vi "MotorCommand.vi"() -> ()   [LabVIEW 2010]
panel:
  out "Value 8":u16=1000
  in  "Enable 8":bool
  in  "Motor 8":u16(slide)=1000 min=1000 max=2000 scale=1000.0..2000.0
  out "Value 7":u16=1000
  in  "Enable 7":bool
  in  "Motor 7":u16(slide)=1000 min=1000 max=2000 scale=1000.0..2000.0
  out "Value 6":u16=1000
  in  "Enable 6":bool
  in  "Motor 6":u16(slide)=1000 min=1000 max=2000 scale=1000.0..2000.0
  out "Value 5":u16=1000
  in  "Enable 5":bool
  in  "Motor 5":u16(slide)=1000 min=1000 max=2000 scale=1000.0..2000.0
  out "Value 4":u16=1000
  in  "Enable 4":bool
  in  "Motor 4":u16(slide)=1000 min=1000 max=2000 scale=1000.0..2000.0
  out "Value 3":u16=1000
  in  "Enable 3":bool
  in  "Motor 3":u16(slide)=1000 min=1000 max=2000 scale=1000.0..2000.0
  out "Value 2":u16=1000
  in  "Enable 2":bool
  in  "Motor 2":u16(slide)=1000 min=1000 max=2000 scale=1000.0..2000.0
  out "Value 1":u16=1000
  in  "Enable 1":bool
  in  "Motor 1":u16(slide)=1000 min=1000 max=2000 scale=1000.0..2000.0
  in  "SendCommand":bool
  in  "StopCommand":bool
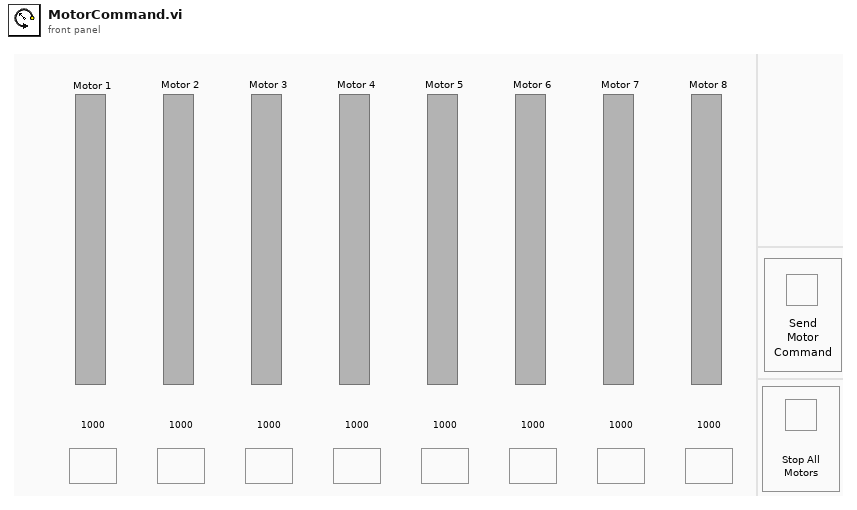
[diagram p1: front panel]
types:
  T1 = cluster{"Error":errorcluster, "GUIQueue":refnum<queue>, "TlmType":string, "NextState":string, "MotorCount":i32, "IniData":string[][]}
  T2 = enum8{"Enabled", "Disabled", "Disabled and Grayed Out"}
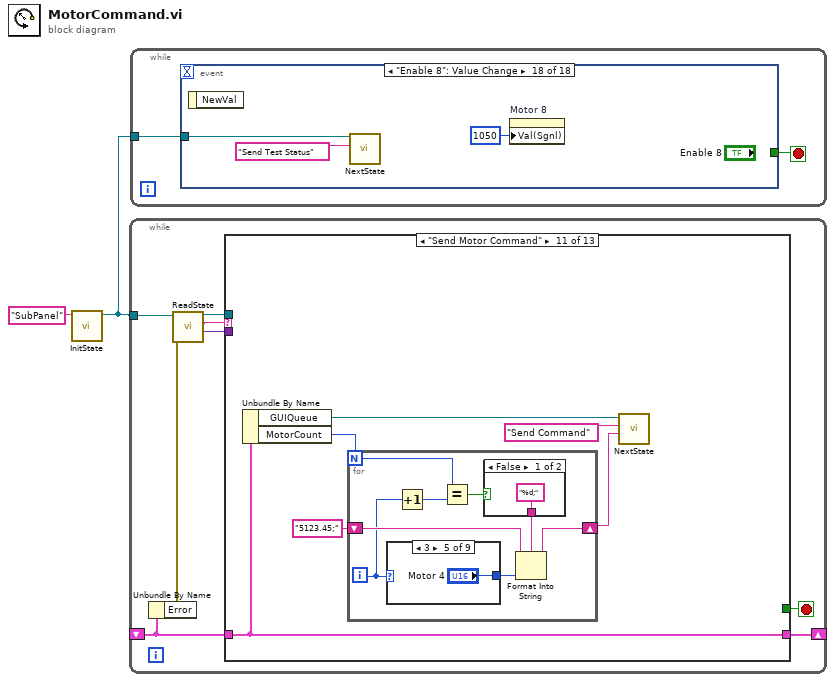
[diagram p0: block diagram]
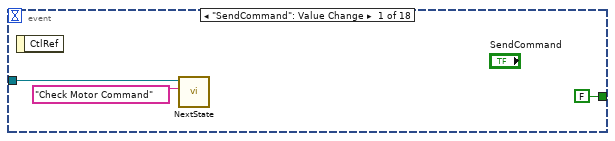
[diagram p2: hidden frame]
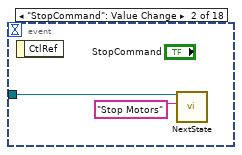
[diagram p3: hidden frame]
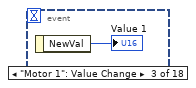
[diagram p4: hidden frame]
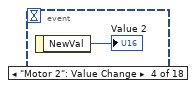
[diagram p5: hidden frame]
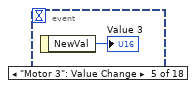
[diagram p6: hidden frame]
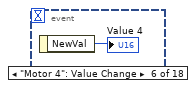
[diagram p7: hidden frame]
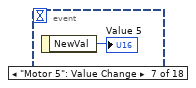
[diagram p8: hidden frame]
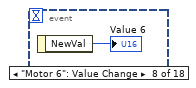
[diagram p9: hidden frame]
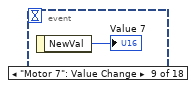
[diagram p10: hidden frame]
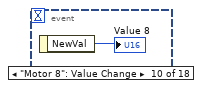
[diagram p11: hidden frame]
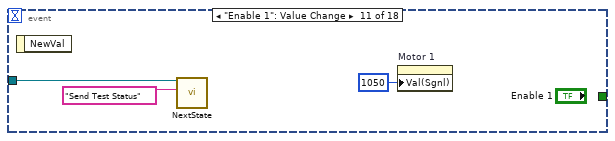
[diagram p12: hidden frame]
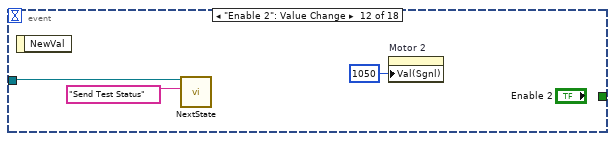
[diagram p13: hidden frame]
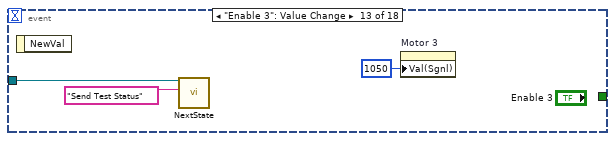
[diagram p14: hidden frame]
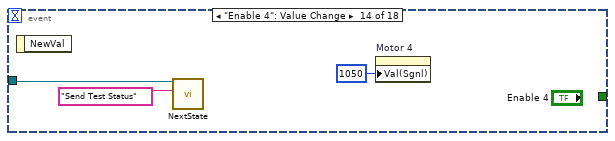
[diagram p15: hidden frame]
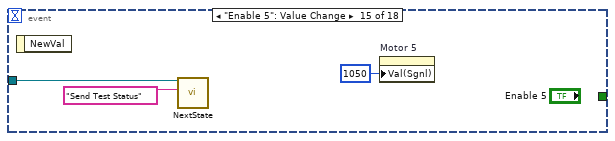
[diagram p16: hidden frame]
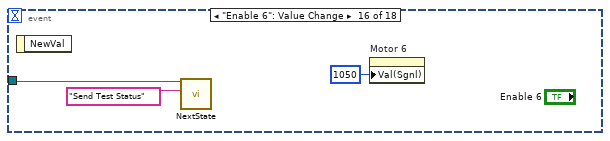
[diagram p17: hidden frame]
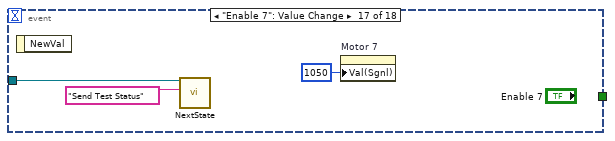
[diagram p18: hidden frame]
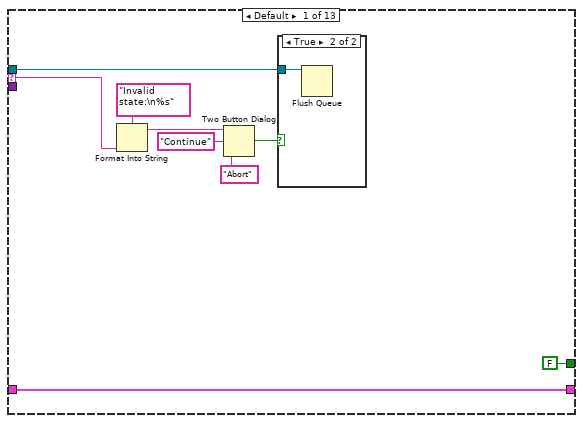
[diagram p19: hidden frame]
diagram:
  n1 = call "InitState.vi"("Name"="SubPanel" ("name (unnamed)")) -> ("Queue Out"=w1:refnum<queue>)  [unwired: 8 in, 1 out]
  n2 = while {
    tunnel: w1 -> [w7]
    shift-right: [w10] -> _
    shift-left: _ -> [w9]
    stop <- w8 stop-if-true
    n3 = Unbundle By Name(w9) -> ("Error"=w6:errorcluster)
    n4 = call "ReadState.vi"("Error In"=w6, "Queue In"=w7) -> ("Data"=w5:variant, "State"=w4:string, "Queue Out"=w3:refnum<queue>)  [unwired: 6 in, 1 out]
    n5 = case shown="\"Send Motor Command\"" w4 {
      tunnel: w3 -> [w11 _ w26 w35 _ _ _ _ _ w78 _ _ w135]
      selector: w4 -> [w17 _ _ _ _ _ _ _ _ _ _ _ _]
      tunnel: w5 -> [_ _ w27 _ _ w70 _ _ _ _ _ _ _]
      tunnel: [w16 w23 w32 w38 w52 w69 w72 w74 w75 w91 w108 w127 w132] -> w10
      tunnel: w9 -> [w16 w23 _ w39 w52 w69 w72 w74 w75 w91 w108 w127 w132]
      tunnel: [FALSE TRUE _ _ _ _ _ TRUE _ _ _ _ _] -> w8
      frame Default {
        n6 = Format Into String(format string="Invalid state:\n%s", w17) -> (resulting string=w18:string)  [unwired: 2 in, 1 out]
        n7 = Two Button Dialog(message=w18, 1:"Abort" ("F button name (\"Cancel\")"), 2:"Continue" ("T button name (\"OK\")")) -> (T button?=w12:bool)
        n8 = case shown="True" w12 {
          tunnel: w11 -> [_ w20]
          frame False {
          }
          frame True {
            n9 = Flush Queue(queue=w20) -> ()  [unwired: 1 in, 3 out]
          }
        }
      }
      frame "Error" {
        n10 = Unbundle By Name(w23) -> ("Error"=w22:errorcluster)
        n11 = call "ErrorDialog.vi"("error in"=w22) -> ("error out"=w21:errorcluster)  [unwired: 10 in]
        n12 = call <vilib>:"Clear Errors.vi"("error in (no error)"=w21) -> ()  [unwired: 6 in, 1 out]
      }
      frame "Initialize" {
        n13 = call "NextState.vi"("State"="Read Initialization", "Queue In"=w26) -> ()  [unwired: 8 in, 2 out]
        n14 = Variant To Data(Variant=w27, type=string[][] [] ("subarray")) -> (data=w29:string[][])  [unwired: 1 in, 1 out]
        n15 = call "InitState.vi"("Name"="GUI") -> ("Queue Out"=w28:refnum<queue>)  [unwired: 8 in, 1 out]
        n16 = Bundle By Name(cluster=T1 {"Error"={"status"=FALSE, "code"=0, "source"=""}, "GUIQueue"=refnum, "TlmType"="", "NextState"="", "MotorCount"=0, "IniData"=[]}, "IniData"=w29, "GUIQueue"=w28) -> (w32:T1)
      }
      frame "Read Initialization" {
        n17 = Unbundle By Name(w39) -> ("IniData"=w41:string[][])
        n18 = call "NextState.vi"("State"="Update Motor Count", "Queue In"=w35) -> ()  [unwired: 8 in, 2 out]
        n19 = Index Array(array=w41, index (col)=0 ("index (row)")) -> (element=w43:string[])  [unwired: 1 in]
        n20 = for {
          tunnel: w43 -> [w50]
          tunnel: string[] ["Motors"] -> [w46] mode=indexing
          tunnel: w41 -> [w49]
          tunnel: [w45] -> w40 mode=indexing
          n21 = Search 1D Array(1D array=w50, element=w46) -> (index of element=w47:i32)  [unwired: 1 in]
          n22 = Index Array(array=w49, index (row)=w47, index (col)=1 ("disabled index (col)")) -> (element=w45:string)
        }
        n23 = Index Array(array=w40) -> (element=w37:string)  [unwired: 1 in]
        n24 = Decimal String To Number(string=w37) -> (number=w36:i32)  [unwired: 2 in, 1 out]
        n25 = Bundle By Name(cluster=w39, "MotorCount"=w36) -> (w38:T1)
      }
      frame "Update Motor Count" {
        n26 = Unbundle By Name(w52) -> ("MotorCount"=w51:i32)
        n27 = for {
          N: 8 -> [_]
          tunnel: w51 -> [w55]
          i -> [w54]
          n28 = Less?(x=w54, y=w55) -> (x < y?=w59:bool)
          n29 = Select(t=T2."Enabled" ("Disabled"), s=w59, f=T2."Disabled and Grayed Out" ("Disabled")) -> (s? t:f=w58:T2)
          n30 = case shown="0" w54 {
            tunnel: w58 -> [_ w60 w61 w62 w63 w64 w65 w66 w67]
            frame Default {
            }
            frame 0 {
              n31 = property on="Motor 1" class="Slide (strict)"("DisabledEnum"=w60) -> ()  [unwired: 2 in, 2 out]
              n32 = property on="Enable 1" class="Bool"("DisabledEnum"=w60) -> ()  [unwired: 2 in, 2 out]
            }
            frame 1 {
              n33 = property on="Motor 2" class="Slide (strict)"("DisabledEnum"=w61) -> ()  [unwired: 2 in, 2 out]
              n34 = property on="Enable 2" class="Bool"("DisabledEnum"=w61) -> ()  [unwired: 2 in, 2 out]
            }
            frame 2 {
              n35 = property on="Motor 3" class="Slide (strict)"("DisabledEnum"=w62) -> ()  [unwired: 2 in, 2 out]
              n36 = property on="Enable 3" class="Bool"("DisabledEnum"=w62) -> ()  [unwired: 2 in, 2 out]
            }
            frame 3 {
              n37 = property on="Motor 4" class="Slide (strict)"("DisabledEnum"=w63) -> ()  [unwired: 2 in, 2 out]
              n38 = property on="Enable 4" class="Bool"("DisabledEnum"=w63) -> ()  [unwired: 2 in, 2 out]
            }
            frame 4 {
              n39 = property on="Motor 5" class="Slide (strict)"("DisabledEnum"=w64) -> ()  [unwired: 2 in, 2 out]
              n40 = property on="Enable 5" class="Bool"("DisabledEnum"=w64) -> ()  [unwired: 2 in, 2 out]
            }
            frame 5 {
              n41 = property on="Motor 6" class="Slide (strict)"("DisabledEnum"=w65) -> ()  [unwired: 2 in, 2 out]
              n42 = property on="Enable 6" class="Bool"("DisabledEnum"=w65) -> ()  [unwired: 2 in, 2 out]
            }
            frame 6 {
              n43 = property on="Motor 7" class="Slide (strict)"("DisabledEnum"=w66) -> ()  [unwired: 2 in, 2 out]
              n44 = property on="Enable 7" class="Bool"("DisabledEnum"=w66) -> ()  [unwired: 2 in, 2 out]
            }
            frame 7 {
              n45 = property on="Motor 8" class="Slide (strict)"("DisabledEnum"=w67) -> ()  [unwired: 2 in, 2 out]
              n46 = property on="Enable 8" class="Bool"("DisabledEnum"=w67) -> ()  [unwired: 2 in, 2 out]
            }
          }
        }
      }
      frame "Update" {
        n47 = Variant To Data(Variant=w70, type=dbl[][] []) -> ()  [unwired: 1 in, 2 out]
      }
      frame "Temporary" {
        n48 = One Button Dialog(message="This feature under contruction.") -> ()  [unwired: 1 in, 1 out]
      }
      frame "Shutdown" {
      }
      frame "----------" {
      }
      frame "Check Motor Command" {
        n49 = local read "Motor 1"() -> (w90:u16)
        n50 = local read "Motor 2"() -> (w89:u16)
        n51 = local read "Motor 3"() -> (w88:u16)
        n52 = local read "Motor 4"() -> (w87:u16)
        n53 = local read "Motor 5"() -> (w86:u16)
        n54 = local read "Motor 6"() -> (w85:u16)
        n55 = local read "Motor 7"() -> (w84:u16)
        n56 = local read "Motor 8"() -> (w83:u16)
        n57 = Build Array(w90, w89, w88, w87, w86, w85, w84, w83) -> (w82:u16[])
        n58 = Greater?(x=w82, y=u16 1200 ("Motor 8")) -> (0:w80:bool[])
        n59 = Or Array Elements(Boolean array=w80) -> (logical OR=w79:bool)
        n60 = case shown="True" w79 {
          tunnel: w78 -> [w93 w96]
          tunnel: [w93 w95] -> w77
          tunnel: ["Send Motor Command" w94] -> w76
          frame False {
          }
          frame True {
            n61 = Two Button Dialog(message="Warning!\n\nSending a motor command\ngreater than 1200 may cause\nthe AeroQuad to lift off if there\nis a propeller attached to the\nmotor.\n\nAre you sure you wish to continue?") -> (T button?=w97:bool)  [unwired: 2 in]
            n62 = case shown="True" w97 {
              tunnel: w96 -> [w100 w102]
              tunnel: [w100 w102] -> w95
              tunnel: ["Stop Motors" "Send Motor Command"] -> w94
              frame False {
              }
              frame True {
              }
            }
          }
        }
        n63 = call "NextState.vi"("State"=w76, "Queue In"=w77) -> ()  [unwired: 8 in, 2 out]
      }
      frame "Send Motor Command" {
        n64 = Unbundle By Name(w108) -> ("GUIQueue"=w105:refnum<queue>, "MotorCount"=w103:i32)
        n65 = for {
          N: w103 -> [w109]
          shift-right: [w114] -> w104
          shift-left: "5123.45;" -> [w115]
          i -> [w110]
          n66 = case shown="3" w110 {
            tunnel: [_ "Motor 1" "Motor 2" "Motor 3" "Motor 4" "Motor 5" "Motor 6" "Motor 7" "Motor 8"] -> w113
            frame Default {
            }
            frame 0 {
            }
            frame 1 {
            }
            frame 2 {
            }
            frame 3 {
            }
            frame 4 {
            }
            frame 5 {
            }
            frame 6 {
            }
            frame 7 {
            }
          }
          n67 = Increment(x=w110) -> (x+1=w111:i32)
          n68 = Equal?(x=w109, y=w111) -> (x = y?=w112:bool)
          n69 = case shown="False" w112 {
            tunnel: ["%d;" ("format string") "%d;" ("format string")] -> w116
            frame False {
            }
            frame True {
            }
          }
          n70 = Format Into String(format string=w116, initial string=w115, w113) -> (resulting string=w114:string)  [unwired: 1 in, 1 out]
        }
        n71 = call "NextState.vi"("Data"=w104, "State"="Send Command", "Queue In"=w105) -> ()  [unwired: 7 in, 2 out]
      }
      frame "Send Test Status" {
        n72 = Unbundle By Name(w127) -> ("GUIQueue"=w130:refnum<queue>)
        n73 = call "NextState.vi"("Data"="Select \"Send Motor Command\" to send commands to motors." ("State"), "State"="Status", "Queue In"=w130) -> ()  [unwired: 7 in, 2 out]
      }
      frame "Stop Motors" {
        w138 = u16 1000 ("Value (Signaling)")
        n74 = Unbundle By Name(w132) -> ("GUIQueue"=w131:refnum<queue>)
        n75 = property on="Motor 1" class="Slide (strict)"("Val(Sgnl)"=w138) -> (error out=w139:errorcluster)  [unwired: 2 in, 1 out]
        n76 = property on="Motor 3" class="Slide (strict)"(error in=w139, "Val(Sgnl)"=w138) -> (error out=w140:errorcluster)  [unwired: 1 in, 1 out]
        n77 = call "NextState.vi"("Data"="All motors stopped." ("State"), "State"="Status", "Queue In"=w131) -> ()  [unwired: 7 in, 2 out]
        n78 = property on="Motor 5" class="Slide (strict)"(error in=w140, "Val(Sgnl)"=w138) -> (error out=w141:errorcluster)  [unwired: 1 in, 1 out]
        n79 = property on="Motor 7" class="Slide (strict)"(error in=w141, "Val(Sgnl)"=w138) -> (error out=w142:errorcluster)  [unwired: 1 in, 1 out]
        n80 = property on="Motor 2" class="Slide (strict)"(error in=w142, "Val(Sgnl)"=w138) -> (error out=w143:errorcluster)  [unwired: 1 in, 1 out]
        n81 = property on="Motor 4" class="Slide (strict)"(error in=w143, "Val(Sgnl)"=w138) -> (error out=w144:errorcluster)  [unwired: 1 in, 1 out]
        n82 = property on="Motor 6" class="Slide (strict)"(error in=w144, "Val(Sgnl)"=w138) -> (error out=w145:errorcluster)  [unwired: 1 in, 1 out]
        n83 = property on="Motor 8" class="Slide (strict)"(error in=w145, "Val(Sgnl)"=w138) -> (error out=w136:errorcluster)  [unwired: 1 in, 1 out]
        n84 = call "NextState.vi"("Error In"=w136, "State"="Send Motor Command", "Queue In"=w135) -> ()  [unwired: 7 in, 2 out]
      }
    }
  }
  n85 = while {
    tunnel: w1 -> [w147]
    stop <- w146 stop-if-true
    n86 = event shown="[17] \"Enable 8\": Value Change" {
      selector: _ -> [_ _ _ _ _ _ _ _ _ _ _ _ _ _ _ _ _ _]
      dyn-events: _ -> [_ _ _ _ _ _ _ _ _ _ _ _ _ _ _ _ _ _]
      timeout: _ -> [_ _ _ _ _ _ _ _ _ _ _ _ _ _ _ _ _ _]
      tunnel: w147 -> [w149 w152 _ _ _ _ _ _ _ _ w162 w164 w167 w170 w173 w176 w179 w182]
      tunnel: [FALSE _ _ _ _ _ _ _ _ _ _ _ _ _ _ _ _ _] -> w146
      event "SendCommand": Value Change {
        n87 = event-data() -> ()  [unwired: 1 in, 1 out]
        n88 = call "NextState.vi"("State"="Check Motor Command", "Queue In"=w149) -> ()  [unwired: 8 in, 2 out]
      }
      event "StopCommand": Value Change {
        n89 = event-data() -> ()  [unwired: 1 in, 1 out]
        n90 = call "NextState.vi"("State"="Stop Motors", "Queue In"=w152) -> ()  [unwired: 8 in, 2 out]
      }
      event "Motor 1": Value Change {
        n91 = event-data() -> ("NewVal"=→"Value 1":u16)  [unwired: 1 in]
      }
      event "Motor 2": Value Change {
        n92 = event-data() -> ("NewVal"=→"Value 2":u16)  [unwired: 1 in]
      }
      event "Motor 3": Value Change {
        n93 = event-data() -> ("NewVal"=→"Value 3":u16)  [unwired: 1 in]
      }
      event "Motor 4": Value Change {
        n94 = event-data() -> ("NewVal"=→"Value 4":u16)  [unwired: 1 in]
      }
      event "Motor 5": Value Change {
        n95 = event-data() -> ("NewVal"=→"Value 5":u16)  [unwired: 1 in]
      }
      event "Motor 6": Value Change {
        n96 = event-data() -> ("NewVal"=→"Value 6":u16)  [unwired: 1 in]
      }
      event "Motor 7": Value Change {
        n97 = event-data() -> ("NewVal"=→"Value 7":u16)  [unwired: 1 in]
      }
      event "Motor 8": Value Change {
        n98 = event-data() -> ("NewVal"=→"Value 8":u16)  [unwired: 1 in]
      }
      event "Enable 1": Value Change {
        n99 = event-data() -> ()  [unwired: 1 in, 1 out]
        n100 = call "NextState.vi"("State"="Send Test Status", "Queue In"=w162) -> ()  [unwired: 8 in, 2 out]
        n101 = property on="Motor 1" class="Slide (strict)"("Val(Sgnl)"=u16 1050 ("Value (Signaling)")) -> ()  [unwired: 2 in, 2 out]
      }
      event "Enable 2": Value Change {
        n102 = event-data() -> ()  [unwired: 1 in, 1 out]
        n103 = call "NextState.vi"("State"="Send Test Status", "Queue In"=w164) -> ()  [unwired: 8 in, 2 out]
        n104 = property on="Motor 2" class="Slide (strict)"("Val(Sgnl)"=u16 1050 ("Value (Signaling)")) -> ()  [unwired: 2 in, 2 out]
      }
      event "Enable 3": Value Change {
        n105 = event-data() -> ()  [unwired: 1 in, 1 out]
        n106 = call "NextState.vi"("State"="Send Test Status", "Queue In"=w167) -> ()  [unwired: 8 in, 2 out]
        n107 = property on="Motor 3" class="Slide (strict)"("Val(Sgnl)"=u16 1050 ("Value (Signaling)")) -> ()  [unwired: 2 in, 2 out]
      }
      event "Enable 4": Value Change {
        n108 = event-data() -> ()  [unwired: 1 in, 1 out]
        n109 = call "NextState.vi"("State"="Send Test Status", "Queue In"=w170) -> ()  [unwired: 8 in, 2 out]
        n110 = property on="Motor 4" class="Slide (strict)"("Val(Sgnl)"=u16 1050 ("Value (Signaling)")) -> ()  [unwired: 2 in, 2 out]
      }
      event "Enable 5": Value Change {
        n111 = event-data() -> ()  [unwired: 1 in, 1 out]
        n112 = call "NextState.vi"("State"="Send Test Status", "Queue In"=w173) -> ()  [unwired: 8 in, 2 out]
        n113 = property on="Motor 5" class="Slide (strict)"("Val(Sgnl)"=u16 1050 ("Value (Signaling)")) -> ()  [unwired: 2 in, 2 out]
      }
      event "Enable 6": Value Change {
        n114 = event-data() -> ()  [unwired: 1 in, 1 out]
        n115 = call "NextState.vi"("State"="Send Test Status", "Queue In"=w176) -> ()  [unwired: 8 in, 2 out]
        n116 = property on="Motor 6" class="Slide (strict)"("Val(Sgnl)"=u16 1050 ("Value (Signaling)")) -> ()  [unwired: 2 in, 2 out]
      }
      event "Enable 7": Value Change {
        n117 = event-data() -> ()  [unwired: 1 in, 1 out]
        n118 = call "NextState.vi"("State"="Send Test Status", "Queue In"=w179) -> ()  [unwired: 8 in, 2 out]
        n119 = property on="Motor 7" class="Slide (strict)"("Val(Sgnl)"=u16 1050 ("Value (Signaling)")) -> ()  [unwired: 2 in, 2 out]
      }
      event "Enable 8": Value Change {
        n120 = event-data() -> ()  [unwired: 1 in, 1 out]
        n121 = call "NextState.vi"("State"="Send Test Status", "Queue In"=w182) -> ()  [unwired: 8 in, 2 out]
        n122 = property on="Motor 8" class="Slide (strict)"("Val(Sgnl)"=u16 1050 ("Value (Signaling)")) -> ()  [unwired: 2 in, 2 out]
      }
    }
  }
